vi "VBus Set Values.vi"(6 "Rear Right":dbl, 7 "Rear Left":dbl, 8 "error in":errorcluster, 9 "Front Right":dbl, 10 "Front Left":dbl, 11 "RobotDriveDevRef in":T1) -> (0 "error out":errorcluster, 3 "RobotDriveDevRef out":T1)   [LabVIEW 2017, in "MechamunDrive.lvlib"]
uses:
  MechamunDrive.lvlib
  <vilib>/Rock Robotics/WPI/RobotDrive/WPI_RobotDriveDevRef.ctl
  <vilib>/Rock Robotics/WPI/MotorControl/WPI_MotorControlDeviceRef.ctl
  <vilib>/Rock Robotics/WPI/MotorControl/WPI_MotorControlType.ctl
  <vilib>/Rock Robotics/SystemInterfaces/DIO/FPGA_DIOPWMChannel.ctl
  <vilib>/Rock Robotics/WPI/PWM/WPI_PWMDeadband.ctl
  <vilib>/Rock Robotics/SystemInterfaces/DIO/FPGA_DIOChannel.ctl
  <vilib>/Rock Robotics/WPI/RobotDrive/WPI_RobotDriveMotorSelectorEnum.ctl
  <vilib>/Rock Robotics/WPI/RobotDrive/WPI_RobotDriveSafetyCheck.vi
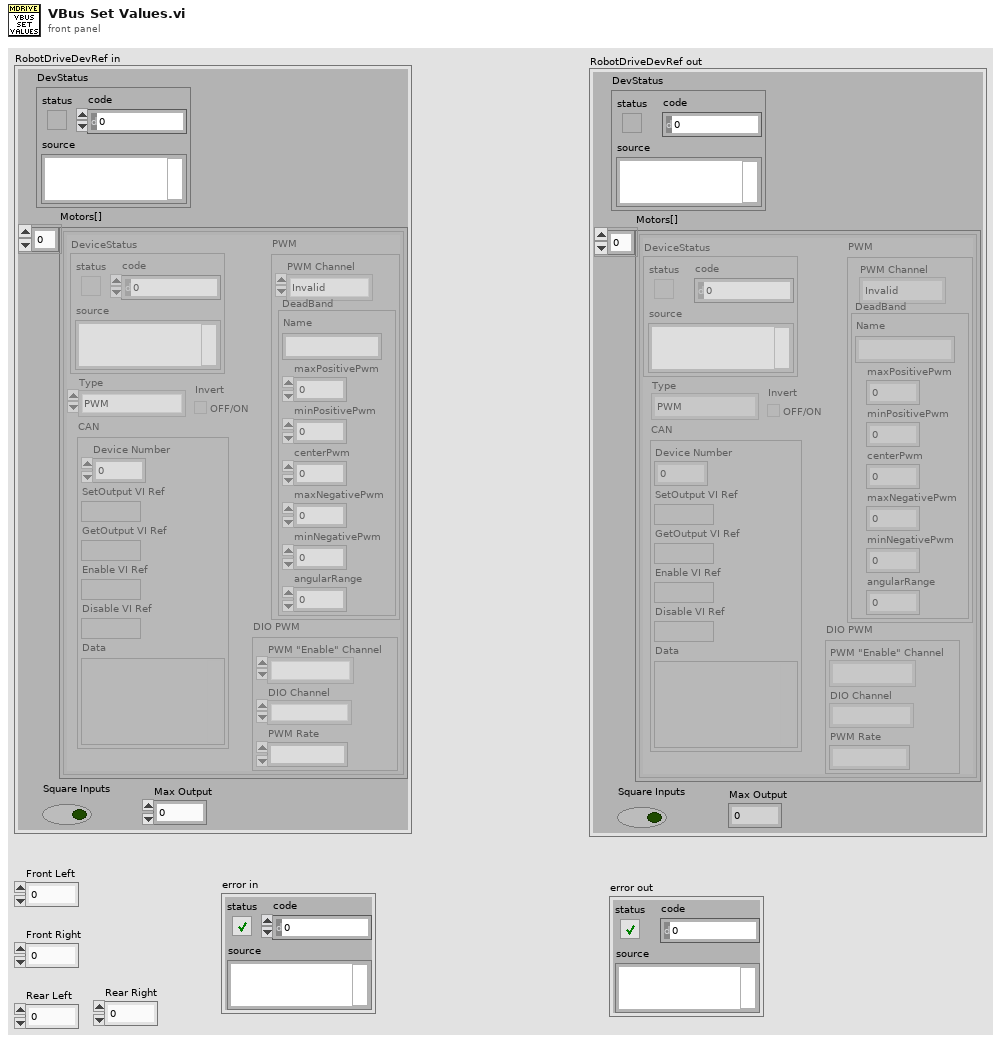
[diagram p1: front panel]
types:
  T1 = typedef "WPI_RobotDriveDevRef.ctl" = cluster{"DevStatus":errorcluster, "Motors[]":T2[], "Square Inputs":bool, "Max Output":dbl}
  T2 = typedef "WPI_MotorControlDeviceRef.ctl" = cluster{"DeviceStatus":errorcluster, "Type":T3, "PWM":cluster{"PWM Channel":T4, "DeadBand":T5}, "CAN":cluster{"Device Number":u8, "SetOutput VI Ref":variant, "GetOutput VI Ref":variant, "Enable VI Ref":variant, "Disable VI Ref":variant, "Data":variant}, "Invert":bool, "DIO PWM":cluster{"PWM \"Enable\" Channel":T4, "DIOChannel":T6, "PWM Rate":dbl}}
  T3 = typedef "WPI_MotorControlType.ctl" = enum16{"PWM", "CAN", "DIO PWM"}
  T4 = typedef "FPGA_DIOPWMChannel.ctl" = enum8{"PWM 0", "PWM 1", "PWM 2", "PWM 3", "PWM 4", "PWM 5", "PWM 6", "PWM 7", "PWM 8", "PWM 9", "PWM MXP 0", "PWM MXP 1", "PWM MXP 2", "PWM MXP 3", "PWM MXP 4", "PWM MXP 5", "PWM MXP 6", "PWM MXP 7", "PWM MXP 8", "PWM MXP 9", "Invalid"}
  T5 = typedef "WPI_PWMDeadband.ctl" = cluster{"Name":string, "maxPositivePwm":i32, "minPositivePwm":i32, "centerPwm":i32, "maxNegativePwm":i32, "minNegativePwm":i32, "angularRange":u16}
  T6 = typedef "FPGA_DIOChannel.ctl" = enum8{"DIO 0", "DIO 1", "DIO 2", "DIO 3", "DIO 4", "DIO 5", "DIO 6", "DIO 7", "DIO 8", "DIO 9", "DIO MXP 0", "DIO MXP 1", "DIO MXP 2", "DIO MXP 3", "DIO MXP 4", "DIO MXP 5", "DIO MXP 6", "DIO MXP 7", "DIO MXP 8", "DIO MXP 9", "DIO MXP 10", "DIO MXP 11", "DIO MXP 12", "DIO MXP 13", "DIO MXP 14", "DIO MXP 15", "SPI Port CS1", "SPI Port CS2", "SPI Port CS3", "SPI Port MISO", "SPI Port MOSI", "Invalid"}
  T7 = typedef "WPI_RobotDriveMotorSelectorEnum.ctl" = enum16{"Rear Left Motor", "Rear Right Motor", "Front Left Motor", "Front Right Motor"}
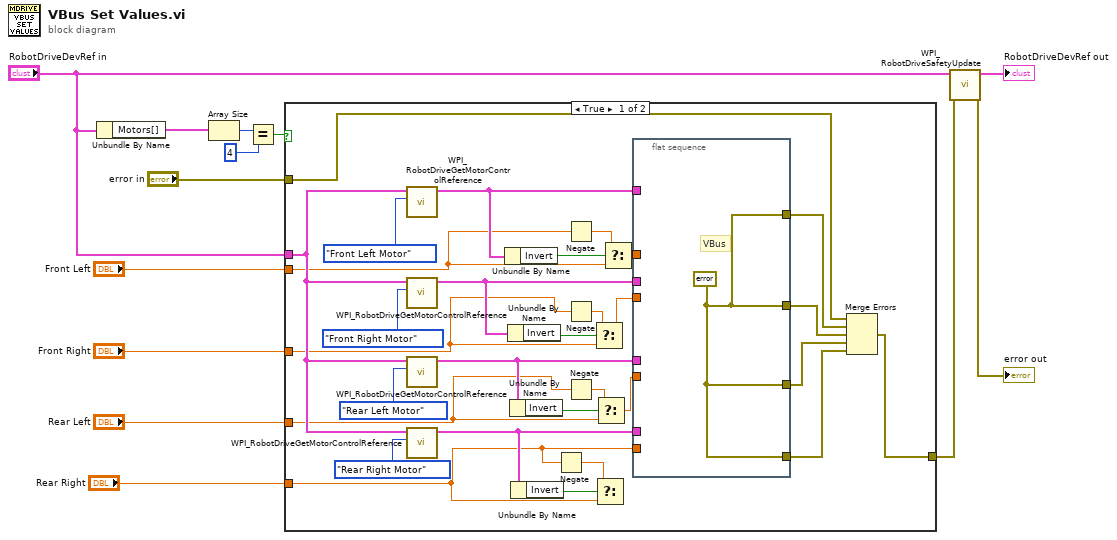
[diagram p0: block diagram]
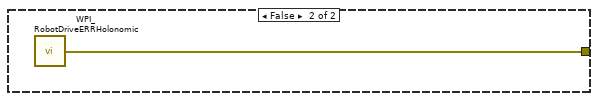
[diagram p2: hidden frame]
diagram:
  n1 = Unbundle By Name("RobotDriveDevRef in") -> ("Motors[]"=w6:T2[])
  n2 = Array Size(array=w6) -> (size(s)=w2:i32)
  n3 = Equal?(x=w2, y=4) -> (x = y?=w4:bool)
  n4 = case shown="True" w4 {
    tunnel: "Front Left" -> [w16 _]
    tunnel: "Front Right" -> [w21 _]
    tunnel: "RobotDriveDevRef in" -> [w39 _]
    tunnel: [w34 w45] -> w5
    tunnel: "Rear Left" -> [w19 _]
    tunnel: "Rear Right" -> [w24 _]
    tunnel: "error in" -> [w14 _]
    frame True {
      n5 = call <vilib>:"WPI_RobotDriveGetMotorControlReference.vi"("MotorIndex"=WPI_RobotDriveMotorSelectorEnum."Front Left Motor", "RobotDriveDevRef"=w39) -> ("MotorControlDeviceRef"=w30:T2)  [unwired: 9 out]
      n6 = call <vilib>:"WPI_RobotDriveGetMotorControlReference.vi"("MotorIndex"=WPI_RobotDriveMotorSelectorEnum."Front Right Motor", "RobotDriveDevRef"=w39) -> ("MotorControlDeviceRef"=w31:T2)  [unwired: 9 out]
      n7 = call <vilib>:"WPI_RobotDriveGetMotorControlReference.vi"("MotorIndex"=WPI_RobotDriveMotorSelectorEnum."Rear Left Motor", "RobotDriveDevRef"=w39) -> ("MotorControlDeviceRef"=w32:T2)  [unwired: 9 out]
      n8 = call <vilib>:"WPI_RobotDriveGetMotorControlReference.vi"("MotorIndex"=WPI_RobotDriveMotorSelectorEnum."Rear Right Motor", "RobotDriveDevRef"=w39) -> ("MotorControlDeviceRef"=w33:T2)  [unwired: 9 out]
      n9 = Unbundle By Name(w30) -> ("Invert"=w28:bool)
      n10 = Unbundle By Name(w31) -> ("Invert"=w27:bool)
      n11 = Unbundle By Name(w32) -> ("Invert"=w26:bool)
      n12 = Unbundle By Name(w33) -> ("Invert"=w29:bool)
      n13 = Negate(x=w24) -> (-x=w25:dbl)
      n14 = Negate(x=w16) -> (-x=w17:dbl)
      n15 = Negate(x=w21) -> (-x=w22:dbl)
      n16 = Negate(x=w19) -> (-x=w23:dbl)
      n17 = Select(t=w22, s=w27, f=w21) -> (s? t:f=w20:dbl)
      n18 = Select(t=w25, s=w29, f=w24) -> ()  [unwired: 1 out]
      n19 = Select(t=w23, s=w26, f=w19) -> (s? t:f=w18:dbl)
      n20 = Select(t=w17, s=w28, f=w16) -> (s? t:f=w15:dbl)
      n21 = flat-sequence {
        tunnel: [w44] -> w38
        tunnel: [w44] -> w37
        tunnel: [w44] -> w36
        tunnel: [w44] -> w35
        tunnel: w33 -> [_]
        tunnel: w32 -> [_]
        tunnel: w31 -> [_]
        tunnel: w30 -> [_]
        tunnel: w24 -> [_]
        tunnel: w20 -> [_]
        tunnel: w18 -> [_]
        tunnel: w15 -> [_]
        frame #0 {
          w44 = errorcluster {"status"=FALSE, "code"=0, "source"=""} ("error out")
          # "VBus"
        }
      }
      n22 = Merge Errors(w14, w35, w36, w37, w38) -> (w34:errorcluster)
    }
    frame False {
      n23 = call <vilib>:"WPI_RobotDriveERRHolonomic.vi"() -> ("error out"=w45:errorcluster)
    }
  }
  n24 = call <vilib>:"WPI_RobotDriveSafetyUpdate.vi"("error in (no error)"=w5, "RobotDriveDevRef"="RobotDriveDevRef in") -> ("error out"=→"error out":errorcluster, "RobotDriveDevRef"=→"RobotDriveDevRef out":T1)  [unwired: 8 out]
